vi "fit_transform.vi"(8 "error in (no error)":errorcluster caption="entrée d'erreur (pas d'erreur)", 11 "MiniBatchKMeans.lvclass 2":refnum<class "MiniBatchKMeans.lvclass">) -> (0 "error out":errorcluster caption="sortie d'erreur", 2 "X_new":dbl[][](array[numeric]), 3 "MiniBatchKMeans.lvclass":refnum<class "MiniBatchKMeans.lvclass">)   [LabVIEW 2020, in "MiniBatchKMeans.lvclass"]
doc: "Compute clustering and transform X to cluster-distance space.\n\n Equivalent to fit(X).transform(X), but more efficiently implemented.\n\n Parameters\n ----------\n X : {array-like, sparse matrix} of shape (n_samples, n_features)\n New data to transform.\n\n y : Ignored\n Not used, present here for API consistency by convention.\n\n sample_weight : array-like of shape (n_samples,), default=None\n The weights for each observation in X. If None, all observations\n are assigned equal weight.\n\n Returns\n -------\n X_new : ndarray of shape (n_samples, n_clusters)\n X transformed in the new space."
uses:
  MiniBatchKMeans.lvclass
  C:/Users/cipop/TDF Dropbox/2_Technologies de France/1 - Services et Etudes/PLAIY/2 - DEV/PLAIYLAB/code/Python/Python.lvclass
  C:/Users/cipop/TDF Dropbox/2_Technologies de France/1 - Services et Etudes/PLAIY/2 - DEV/PLAIYLAB/code/Model/Model.lvclass
  MiniBatchKMeans.lvclass/MiniBatchKMeans.ctl
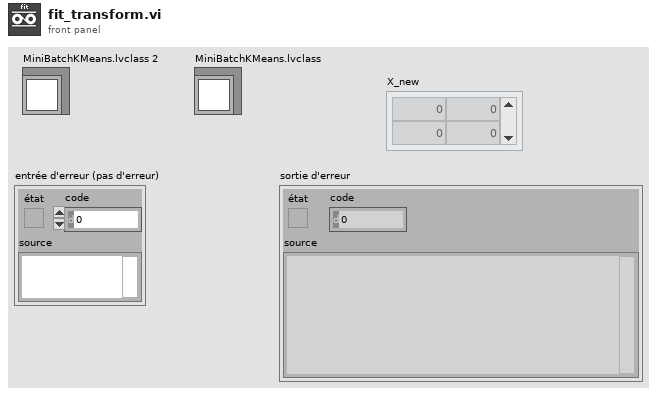
[diagram p1: front panel]
types:
  T1 = typedef "data.ctl" = cluster{"name":string, "X":dbl[][]}
  T2 = typedef "mini_batch_kmeans_data.ctl" = cluster{"sample_weight":dbl[]}
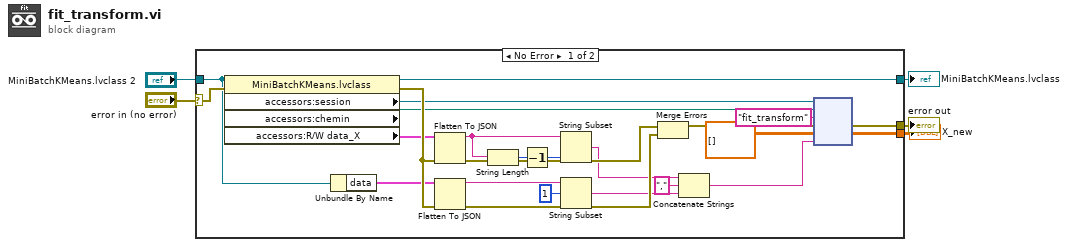
[diagram p0: block diagram]
diagram:
  n1 = case shown="No Error" "error in (no error)" {
    selector: "error in (no error)" -> [w27 w31]
    tunnel: [w28 w31] -> w4
    tunnel: [w10 w30] -> w2
    tunnel: "MiniBatchKMeans.lvclass 2" -> [w9 w30]
    tunnel: [w6 _] -> w1
    frame No Error {
      n2 = property class="MiniBatchKMeans.lvclass"(reference=w9, error in=w27) -> (reference out=w10:refnum<class "MiniBatchKMeans.lvclass">, error out=w23:errorcluster, "accessors:session"=w13:refnum<k35>, "accessors:chemin"=w12:path, "accessors:R/W data_X"=w14:T1)
      n3 = Unbundle By Name(w9) -> ("data"=w8:T2)
      n4 = Flatten To JSON(anything=w14, error in (no error)=w23) -> (JSON string=w24:string, 11:w19:errorcluster)  [unwired: 1 in]
      n5 = Flatten To JSON(anything=w8, error in (no error)=w23) -> (JSON string=w21:string, 11:w20:errorcluster)  [unwired: 1 in]
      n6 = String Length(string=w24) -> (length=w26:i32)
      n7 = Decrement(x=w26) -> (x-1=w25:i32)
      n8 = String Subset(string=w24, length (rest)=w25) -> (substring=w17:string)  [unwired: 1 in]
      n9 = String Subset(string=w21, offset (0)=1) -> (substring=w16:string)  [unwired: 1 in]
      n10 = Merge Errors(w19, w20) -> (w11:errorcluster)
      n11 = Concatenate Strings(w17, "," ("string"), w16) -> (w15:string)
      n12 = node(w13, w12, "fit_transform" ("nom de la fonction"), w11, dbl[][] [], w15) -> (w28:errorcluster, w6:dbl[][])  [unwired: 1 in, 3 out]
    }
    frame Error {
    }
  }
  "error out" <- w4
  "MiniBatchKMeans.lvclass" <- w2
  "X_new" <- w1
